vi "Denoising with Wavelet (Basic).vi"() -> ()   [LabVIEW 2023]
doc: "This example shows how to reduce noise of an image with the WA Denoise VI. The flower image is contaminated by some Gaussian white noise with a standard deviation 5. This example uses the undecimated wavelet transform-based method to denoise the image.\n\n<b>Instructions:</b>\n1) Run this VI.\n2) Compare the noisy image and denoised image with different settings."
uses:
  Images/_Images.ctl
  <vilib>/vision/NI_Vision_Development_Module.lvlib
  <vilib>/addons/_Advanced Signal Processing/NI_AdvSigProcWA.lvlib
panel:
  in  "Image Selector":T1=enum."Connector1"
  out "diff":T2(plugin-control)
  out "Image 2":T2(plugin-control)
  out "Image":T2(plugin-control)
  in  "Threshold settings":T3={"Thresholding Rule"=enum."SURE", "Rescaling Method"=enum."Single level", "Soft Threshold?"=TRUE}
  in  "Wavelet":u16(ring) items=["db02"=0, "db03"=1, "db04"=2, "db05"=3, "db06"=4, "db07"=5, "db08"=6, "db09"=7, "db10"=8, "db11"=9, "db12"=10, "db13"=11, "db14"=12, "Haar"=13, "bior1_3"=14, "bior1_5"=15, "bior2_2"=16, "bior2_4"=17, "bior2_6"=18, "bior2_8"=19, "bior3_1"=20, "bior3_3"=21, "bior3_5"=22, "bior3_7"=23, "bior3_9"=24, "bior4_4 (FBI)"=25, "bior5_5"=38, "bior6_8"=39, "coif1"=26, "coif2"=27, "coif3"=28, "coif4"=29, "coif5"=30, "sym2"=31, "sym3"=32, "sym4"=33, "sym5"=34, "sym6"=35, "sym7"=36, "sym8"=37]
  in  "Levels":i32=4
  # "Denoises the image by using undecimated wavelet transform"
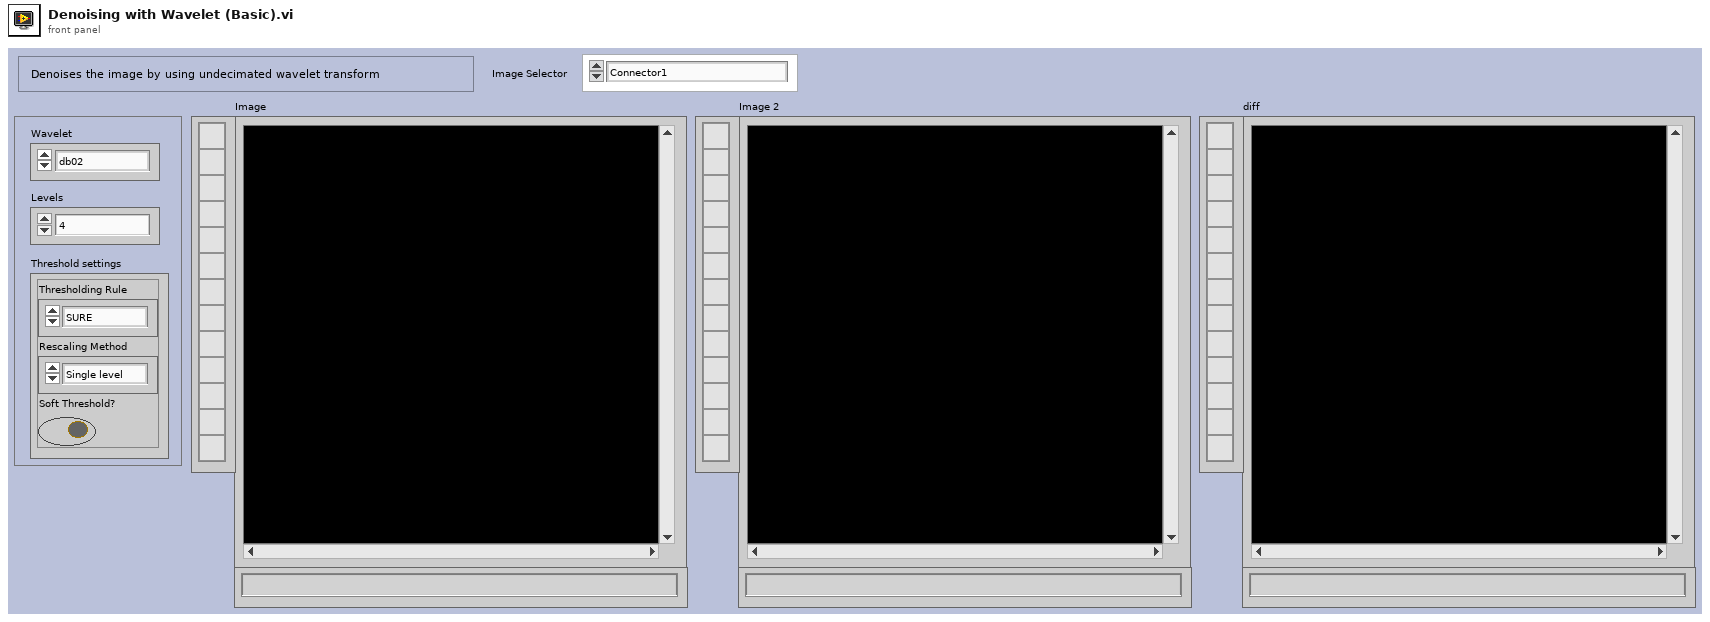
[diagram p1: front panel]
types:
  T1 = typedef "_Images.ctl" = enum16{"Balls2", "Battery1", "Battery2", "Connector1", "Subwoofer1", "Subwoofer2", "Subwoofer3", "Subwoofer4", "Hase1", "Lamp1", "Lamp2", "Mouse1", "PhotoLens1", "Po1", "PowerSupply1", "Router", "--- Step Wedges ---", "Stepwedge1", "Stepwedge2", "Stepwedge3", "--- Fusion ---", "Fusion160kV", "Fusion2-120kV", "Fusion2-320kV", "Fusion300kV", "FusionPart1-120kV", "FusionPart1-180kV", "--- PART 01 ---", "Part1", "Part2", "Part3", "Part4", "Part5", "Part6", "Part7", "Part8", "--- Different Integrations ---", "Step2737-02Int", "Step2737-04Int", "Step2737-08Int", "Step2737-16Int", "Step2737-32Int", "Step2737-64Int"}
  T2 = typedef "IMAQ Image.ctl" = refnum<image>
  T3 = cluster{"Thresholding Rule":enum16{"SURE", "Hybrid", "Universal", "Minimax"}, "Rescaling Method":enum16{"One", "Single level", "Multiple levels"}, "Soft Threshold?":bool}
  T4 = typedef "Image Type" = u32
  T5 = cluster{"low_low":dbl[][], "low_high":dbl[][], "high_low":dbl[][], "high_high":dbl[][]}[]
  T6 = cluster{"low_low":dbl[][], "signal shrinkage":dbl[][], "signal shrinkage":dbl[][], "signal shrinkage":dbl[][]}
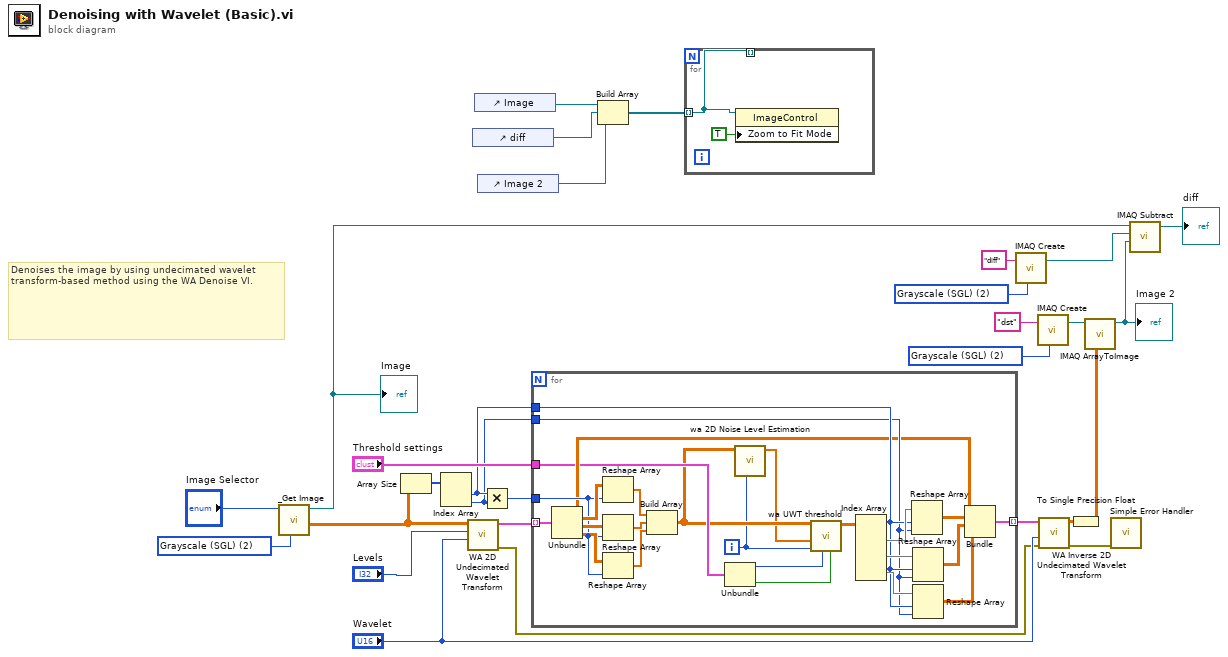
[diagram p0: block diagram]
diagram:
  w22 = T4 2 items=["Grayscale (U8)", "Grayscale (I16)", "Grayscale (SGL)", "Complex (CSG)", "RGB (U32)", "HSL (U32)", "RGB (U64)", "Grayscale (U16)"] ("Image Type")
  w25 = T4 2 items=["Grayscale (U8)", "Grayscale (I16)", "Grayscale (SGL)", "Complex (CSG)", "RGB (U32)", "HSL (U32)", "RGB (U64)", "Grayscale (U16)"] ("Image Type")
  w28 = T4 2 items=["Grayscale (U8)", "Grayscale (I16)", "Grayscale (SGL)", "Complex (CSG)", "RGB (U32)", "HSL (U32)", "RGB (U64)", "Grayscale (U16)"] ("Image Type (U16)")
  # "Denoises the image by using undecimated wavelet transform-based method using the WA Denoise VI."
  n1 = call "_Get Image.vi"("Image Type (U16)"=w28, "Image"="Image Selector") -> ("Image Pixels (Float)"=w17:dbl[][], "Image Out"=w21:T2)  [unwired: 6 in, 2 out]
  "Image" <- w21
  n2 = Array Size(array=w17) -> (size(s)=w10:i32[])
  n3 = Index Array(array=w10) -> (element #1=w8:i32, element #2=w7:i32)  [unwired: 2 in]
  n4 = call <vilib>:"WA 2D Undecimated Wavelet Transform.vi"("wavelet"="Wavelet", "levels"="Levels", "signal"=w17) -> ("error out"=w6:errorcluster, "UWT coef"=w11:T5)  [unwired: 2 in, 5 out]
  n5 = control-ref of="diff"() -> (w3:refnum<vi>)
  n6 = control-ref of="Image"() -> (w4:refnum<vi>)
  n7 = control-ref of="Image 2"() -> (w2:refnum<vi>)
  n8 = Multiply(x=w8, y=w7) -> (x*y=w9:i32)
  n9 = for {
    tunnel: "Threshold settings" -> [w36]
    tunnel: w11 -> [w54] mode=indexing
    tunnel: w9 -> [w47]
    tunnel: w8 -> [w43]
    tunnel: w7 -> [w42]
    tunnel: [w37] -> w5 mode=indexing
    i -> [w33]
    n10 = Unbundle(w54) -> ("low_low"=w41:dbl[][], "low_high"=w53:dbl[][], "high_low"=w51:dbl[][], "high_high"=w49:dbl[][])
    n11 = Reshape Array(w53, w47) -> (w52:dbl[])
    n12 = Reshape Array(w51, w47) -> (w50:dbl[])
    n13 = Reshape Array(w49, w47) -> (w48:dbl[])
    n14 = Build Array(w52, w50, w48) -> (w35:dbl[][])
    n15 = Unbundle(w36) -> ("Thresholding Rule"=w32:enum16{"SURE", "Hybrid", "Universal", "Minimax"}, "Soft Threshold?"=w31:bool)  [unwired: 1 out]
    n16 = call <vilib>:"wa 2D Noise Level Estimation.vi"("level id"=w33, "UWT"=w35) -> ("noise level out"=w34:dbl[])  [unwired: 2 in, 7 out]
    n17 = call <vilib>:"wa UWT threshold.vi"("soft threshold?"=w31, "thresholding rule"=w32, "level id"=w33, "noise level out"=w34, "UWT coef"=w35) -> ("signal shrinkage"=w30:dbl[][])  [unwired: 1 in, 5 out]
    n18 = Index Array(array=w30) -> (element #1=w46:dbl[], element #2=w45:dbl[], element #3=w44:dbl[])  [unwired: 6 in]
    n19 = Reshape Array(w46, w43, w42) -> (w40:dbl[][])
    n20 = Reshape Array(w45, w43, w42) -> (w39:dbl[][])
    n21 = Reshape Array(w44, w43, w42) -> (w38:dbl[][])
    n22 = Bundle("low_low"=w41, "signal shrinkage"=w40, "signal shrinkage"=w39, "signal shrinkage"=w38) -> (w37:T6)  [unwired: 1 out]
  }
  n23 = Build Array(w4, w3, w2) -> (w1:refnum<vi>[])
  n24 = for {
    tunnel: w1 -> [w56] mode=indexing
    tunnel: [w56] -> _ mode=indexing
    n25 = property class="ImageControl"(reference=w56, "Zoom to Fit Mode"=TRUE) -> ()  [unwired: 1 in, 2 out]
  }
  n26 = call "IMAQ Create"("Image Name"="diff", "Image Type"=w22) -> ("New Image"=w19:T2)  [unwired: 3 in, 1 out]
  n27 = call "IMAQ Create"("Image Name"="dst", "Image Type"=w25) -> ("New Image"=w26:T2)  [unwired: 3 in, 1 out]
  n28 = call <vilib>:"WA Inverse 2D Undecimated Wavelet Transform.vi"("error in (no error)"=w6, "wavelet"="Wavelet", "UWT coef"=w5) -> ("error out"=w12:errorcluster, "signal"=w16:dbl[][])  [unwired: 1 in, 6 out]
  n29 = To Single Precision Float(number=w16) -> (single precision float=w24:sgl[][])
  n30 = call "IMAQ ArrayToImage"("Image Pixels (Float)"=w24, "Image"=w26) -> ("Image Out"=w20:T2)  [unwired: 8 in, 1 out]
  "Image 2" <- w20
  n31 = call <vilib>:"Simple Error Handler.vi"("error in (no error)"=w12) -> ()  [unwired: 4 in, 5 out]
  n32 = call "IMAQ Subtract"("Image Src A"=w21, "Image Dst"=w19, "Image Src B"=w20) -> ("Image Dst Out"=→"diff":T2)  [unwired: 4 in, 1 out]
